vi "TextControlledInstrumControlChangedSub.vi"(2 "Command Array":string[](array[string]), 3 "timeout in ms (1000ms)":i32=1000, 5 "OldVal":variant, 7 "NewVal":variant, 9 "IO Queue":refnum<queue>) -> ()   [LabVIEW 2021]
uses:
  TextControlledInstrumIOQueuePacket.ctl
  <vilib>/Utility/Data Type/NI_Data Type.lvlib
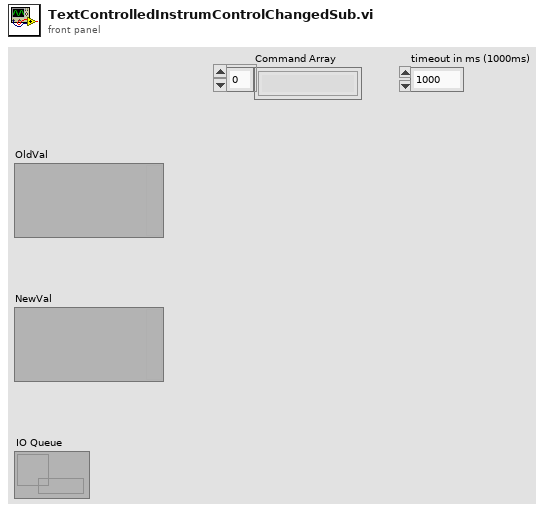
[diagram p1: front panel]
types:
  T1 = typedef "NI_Data Type.lvlib/Data Type.ctl" = enum8{"Invalid Type", "Void", "I8", "I16", "I32", "I64", "U8", "U16", "U32", "U64", "Single Float", "Double Float", "Extended Float", "Single Complex", "Double Complex", "Extended Complex", "Enum U8", "Enum U16", "Enum U32", "Enum U64", "Single Float With Unit", "Double Float With Unit", "Extended Float With Unit", "Single Complex with Unit", "Double Complex with Unit", "Extended Complex with Unit", "Boolean", "String", "Path", "Picture", "Tag", "Array", "Cluster", "Variant", "LV Variant", "Waveform", "Timestamp", "Digital Waveform", "Digital Data", "ExpressData", "Refnum", "External Data", "VI", "Poly VI", "LabVIEW Class Instance", "Fixed Point", "Set Collection", "Map Collection"}
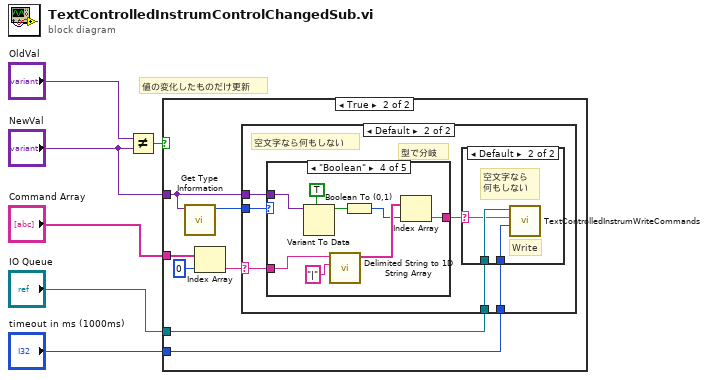
[diagram p0: block diagram]
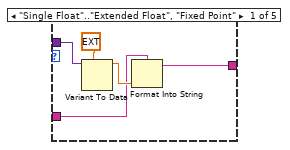
[diagram p5: hidden frame]
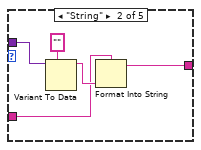
[diagram p6: hidden frame]
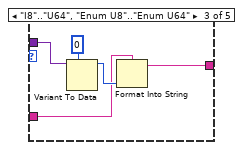
[diagram p7: hidden frame]
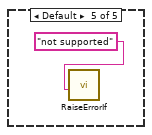
[diagram p8: hidden frame]
diagram:
  # "値の変化したものだけ更新"
  n1 = Not Equal?(x="OldVal", y="NewVal") -> (x != y?=w3:bool)
  n2 = case shown="True" w3 {
    tunnel: "NewVal" -> [_ w11]
    tunnel: "IO Queue" -> [_ w10]
    tunnel: "timeout in ms (1000ms)" -> [_ w9]
    tunnel: "Command Array" -> [_ w8]
    frame False {
    }
    frame True {
      n3 = call <vilib>:"Get Type Information.vi"("variant"=w11) -> ("type"=w13:T1)  [unwired: 6 in, 4 out]
      n4 = Index Array(array=w8, index=0 ("index (row)")) -> (element=w7:string)
      n5 = case shown="Default" w7 {
        selector: w7 -> [_ w15]
        tunnel: w13 -> [_ w19]
        tunnel: w11 -> [_ w18]
        tunnel: w10 -> [_ w17]
        tunnel: w9 -> [_ w16]
        frame "" {
        }
        frame Default {
          # "型で分岐"
          # "空文字なら何もしない"
          n6 = case shown="\"Boolean\"" w19 {
            tunnel: w18 -> [w27 w32 w37 w43 _]
            tunnel: w15 -> [w23 w28 w33 w45 _]
            tunnel: [w24 w30 w35 w38 _] -> w14
            frame "Single Float".."Extended Float", "Fixed Point" {
              n7 = Variant To Data(type=ext 0.0, Variant=w27) -> (data=w25:ext)  [unwired: 1 in, 1 out]
              n8 = Format Into String(format string=w23, w25) -> (resulting string=w24:string)  [unwired: 2 in, 1 out]
            }
            frame "String" {
              n9 = Variant To Data(type="", Variant=w32) -> (data=w31:string)  [unwired: 1 in, 1 out]
              n10 = Format Into String(format string=w28, w31) -> (resulting string=w30:string)  [unwired: 2 in, 1 out]
            }
            frame "I8".."U64", "Enum U8".."Enum U64" {
              n11 = Variant To Data(type=i64 0, Variant=w37) -> (data=w36:i64)  [unwired: 1 in, 1 out]
              n12 = Format Into String(format string=w33, w36) -> (resulting string=w35:string)  [unwired: 2 in, 1 out]
            }
            frame "Boolean" {
              n13 = Variant To Data(type=TRUE, Variant=w43) -> (data=w41:bool)  [unwired: 1 in, 1 out]
              n14 = call <vilib>:"Delimited String to 1D String Array.vi"("delimiter"="|", "delimited string"=w45) -> ("string array"=w40:string[])  [unwired: 9 in]
              n15 = Boolean To (0,1)(Boolean=w41) -> (0, 1=w39:i16)
              n16 = Index Array(array=w40, index=w39) -> (element=w38:string)
            }
            frame Default {
              n17 = call "RaiseErrorIf.vi"("error message"="not supported" ("error source (\" \")")) -> ()  [unwired: 10 in, 1 out]
            }
          }
          n18 = case shown="Default" w14 {
            selector: w14 -> [_ w21]
            tunnel: w17 -> [_ w22]
            tunnel: w16 -> [_ w20]
            frame "" {
            }
            frame Default {
              # "Write"
              # "空文字なら\n何もしない"
              n19 = call "TextControlledInstrumWriteCommands.vi"("timeout in ms (100)"=w20, "Multi-line String"=w21, "IO Queue"=w22) -> ()  [unwired: 7 in, 2 out]
            }
          }
        }
      }
    }
  }
